vi "Get Zernike Coefficients 2.vi"(8 "error in (no error)":errorcluster, 9 "Pupil":cluster{"center":T2, "radius":sgl}, 10 "PupilDetectionOption":T1, 11 "HasoSlopes in":refnum<class "HasoSlopes.lvclass">) -> (0 "error out":errorcluster, 1 "Pupil out":cluster{"center":T2, "radius":sgl}, 2 "Zernike Coefficients":dbl[](array[numeric]), 3 "HasoSlopes out":refnum<class "HasoSlopes.lvclass">)   [LabVIEW 2020]
uses:
  WaveKit/Controls/Point2Df.ctl
  WaveKit/Controls/CircularPupilDetectionParams.ctl
  WaveKit/Controls/PupilDetectionOption.ctl
  WaveKit/Controls/CircularAutoDetectionOptions.ctl
  WaveKit/Controls/PupilDetectionMode.ctl
  WaveKit/Classes/HasoSlopes/HasoSlopes.lvclass
  WaveKit/Classes/ComputePhaseSet/ComputePhaseSet.lvclass
  WaveKit/Classes/Pupil/Pupil.lvclass
  WaveKit/Controls/ZernikeModalPrefs.ctl
  WaveKit/Controls/ZernikeProjectionPupilSetup.ctl
  WaveKit/Classes/ModalCoef/ModalCoef.lvclass
  WaveKit/Controls/WavefrontReconstructionMode.ctl
  WaveKit/Controls/WavefrontModalReconstructionType.ctl
  WaveKit/Classes/HasoData/HasoData.lvclass
panel:
  in  "CircularPupilDetectionParams":T3={"PupilDetectionOption"=enum."Automatic", "AutoDetectionOption"=enum."auto_radius_auto_center", "PupilDetectionMode"=enum."inscribed", "CentralOccultationDetection"=FALSE}
  out "radius":sgl
  out "center":T2
  out "Zernike pupil":i32[][](graph)
  out "Measured pupil":i32[][](graph)
  # "21.9945"
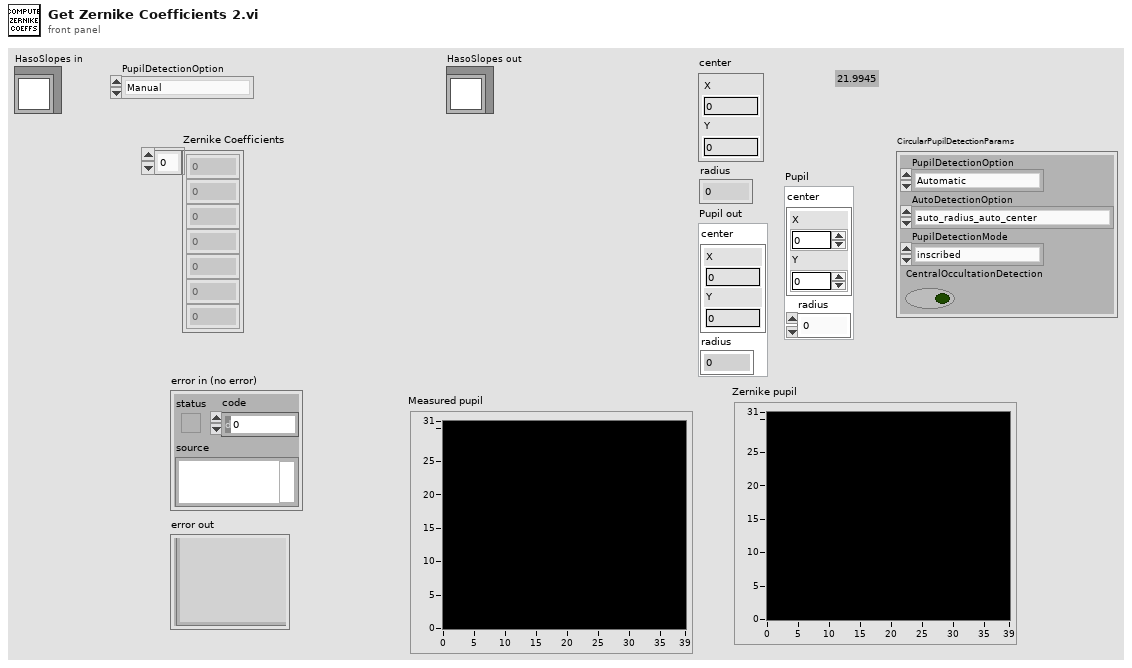
[diagram p1: front panel]
types:
  T1 = typedef "PupilDetectionOption.ctl" = enum16{"Manual", "Automatic"}
  T2 = typedef "Point2Df.ctl" = cluster{"X":sgl, "Y":sgl}
  T3 = typedef "CircularPupilDetectionParams.ctl" = cluster{"PupilDetectionOption":T1, "AutoDetectionOption":T4, "PupilDetectionMode":T5, "CentralOccultationDetection":bool}
  T4 = typedef "CircularAutoDetectionOptions.ctl" = enum16{"manual_radius_auto_center", "manual_center_auto_radius", "auto_radius_auto_center"}
  T5 = typedef "PupilDetectionMode.ctl" = enum16{"inscribed", "circumscribed"}
  T6 = typedef "WavefrontModalReconstructionType.ctl" = enum16{"Legendre", "Zernike"}
  T7 = typedef "WavefrontReconstructionMode.ctl" = enum16{"None", "Modal_Legendre", "Modal_Zernike", "Zonal", "Modal_Zonal_Zernike", "Modal_Zonal_Legendre"}
  T8 = typedef "ZernikeModalPrefs.ctl" = cluster{"Number of coefficients":u32, "Filtered coefficients":u32[], "RMS Zernike normalization":bool, "CircularProjectionPupilDimensions":T9}
  T9 = typedef "ZernikeProjectionPupilSetup.ctl" = cluster{"Pupil center_sspp":T2, "Pupil radius_sspp":sgl}
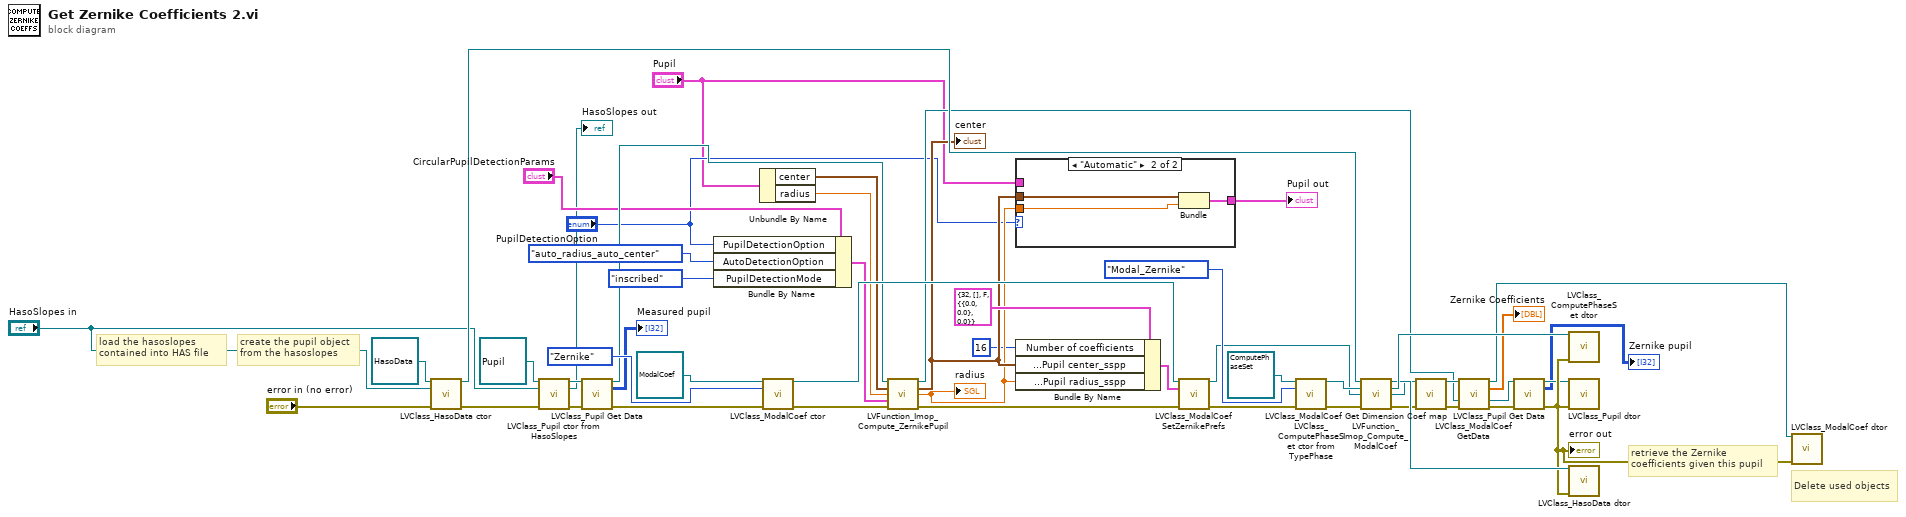
[diagram p0: block diagram]
diagram:
  # "Delete used objects"
  # "retrieve the Zernike\ncoefficients given this pupil"
  # "create the pupil object\nfrom the hasoslopes"
  # "load the hasoslopes\ncontained into HAS file"
  n1 = call "LVClass_HasoData ctor.vi"("HasoData (const)"=refnum<class "HasoData.lvclass"> refnum ("HasoData in"), "HasoSlopes"="HasoSlopes in", "error in (no error)"="error in (no error)") -> ("HasoData (new)"=w33:refnum<class "HasoData.lvclass">, "error out"=w31:errorcluster)  [unwired: 10 in, 1 out]
  n2 = call "LVClass_Pupil ctor from HasoSlopes.vi"("Pupil (const)"=refnum<class "Pupil.lvclass"> refnum ("Pupil in"), "HasoSlopes"="HasoSlopes in", "error in (no error)"=w31) -> ("Pupil (new)"=w29:refnum<class "Pupil.lvclass">, "HasoSlopes (dup)"=→"HasoSlopes out":refnum<class "HasoSlopes.lvclass">, "error out"=w27:errorcluster)  [unwired: 10 in]
  n3 = call "LVClass_Pupil Get Data.vi"("Pupil in"=w29, "error in (no error)"=w27) -> ("Pupil out"=w28:refnum<class "Pupil.lvclass">, "Data"=→"Measured pupil":i32[][], "error out"=w18:errorcluster)  [unwired: 11 in]
  n4 = Bundle By Name(cluster="CircularPupilDetectionParams", "PupilDetectionOption"="PupilDetectionOption", "AutoDetectionOption"=CircularAutoDetectionOptions."auto_radius_auto_center", "PupilDetectionMode"=PupilDetectionMode."inscribed") -> (w8:T3)
  n5 = Unbundle By Name("Pupil") -> ("center"=w15:T2, "radius"=w14:sgl)
  n6 = call "LVClass_ModalCoef ctor.vi"("ModalCoef (const)"=refnum<class "ModalCoef.lvclass"> refnum ("ModalCoef in"), "TypePhase"=WavefrontModalReconstructionType."Zernike", "error in (no error)"=w18) -> ("ModalCoef (new)"=w35:refnum<class "ModalCoef.lvclass">, "error out"=w30:errorcluster)  [unwired: 11 in]
  n7 = call "LVFunction_Imop_Compute_ZernikePupil.vi"("Pupil.lvclass"=w28, "center in"=w15, "radius in"=w14, "CircularPupilDetectionParams"=w8, "error in"=w30) -> ("Pupil.lvclass"=w24:refnum<class "Pupil.lvclass">, "center"=w13:T2, "radius"=w12:sgl, "error out"=w25:errorcluster)  [unwired: 7 in]
  "center" <- w13
  "radius" <- w12
  n8 = case shown="\"Automatic\"" "PupilDetectionOption" {
    tunnel: w13 -> [_ w55]
    tunnel: w12 -> [_ w54]
    tunnel: [w52 w53] -> w11
    tunnel: "Pupil" -> [w52 _]
    frame "Manual", Default {
    }
    frame "Automatic" {
      n9 = Bundle("center"=w55, "radius"=w54) -> (w53:cluster{"center":T2, "radius":sgl})  [unwired: 1 in]
    }
  }
  "Pupil out" <- w11
  n10 = Bundle By Name(cluster=T8 {"Number of coefficients"=32, "Filtered coefficients"=[], "RMS Zernike normalization"=FALSE, "CircularProjectionPupilDimensions"={"Pupil center_sspp"={"X"=0.0, "Y"=0.0}, "Pupil radius_sspp"=0.0}} ("ZernikeModalPrefs"), "Number of coefficients"=u32 16, "CircularProjectionPupilDimensions.Pupil center_sspp"=w13, "CircularProjectionPupilDimensions.Pupil radius_sspp"=w12) -> (w41:T8)
  n11 = call "LVClass_ModalCoef SetZernikePrefs.vi"("ModalCoef in"=w35, "ZernikeModalPrefs"=w41, "error in (no error)"=w25) -> ("ModalCoef out"=w36:refnum<class "ModalCoef.lvclass">, "error out"=w17:errorcluster)  [unwired: 11 in]
  n12 = call "LVClass_ComputePhaseSet ctor from TypePhase.vi"("ComputePhaseSet (const)"=refnum<class "ComputePhaseSet.lvclass"> refnum ("ComputePhaseSet in"), "TypePhase"=WavefrontReconstructionMode."Modal_Zernike", "error in (no error)"=w17) -> ("ComputePhaseSet (new)"=w37:refnum<class "ComputePhaseSet.lvclass">, "error out"=w16:errorcluster)  [unwired: 11 in]
  n13 = call "LVFunction_Imop_Compute_ModalCoef.vi"("HasoData.lvclass"=w33, "ComputePhaseSet.lvclass"=w37, "ModalCoef.lvclass"=w36, "error constant"=w16) -> ("HasoData.lvclass (dup)"=w46:refnum<class "HasoData.lvclass">, "ComputePhaseSet.lvclass (dup)"=w47:refnum<class "ComputePhaseSet.lvclass">, "ModalCoef.lvclass (dup)"=w32:refnum<class "ModalCoef.lvclass">, "error out"=w43:errorcluster)  [unwired: 8 in]
  n14 = call "LVClass_ModalCoef Get Dimension Coef map.vi"("ModalCoef in"=w32, "error in (no error)"=w43) -> ("ModalCoef out"=w48:refnum<class "ModalCoef.lvclass">, "error out"=w44:errorcluster)  [unwired: 11 in, 1 out]
  n15 = call "LVClass_ModalCoef GetData.vi"("ModalCoef in"=w48, "Pupil.lvclass"=w24, "error in (no error)"=w44) -> ("ModalCoef out"=w45:refnum<class "ModalCoef.lvclass">, "coef"=→"Zernike Coefficients":sgl[], "Pupil.lvclass (dup)"=w23:refnum<class "Pupil.lvclass">, "error out"=w22:errorcluster)  [unwired: 8 in, 1 out]
  n16 = call "LVClass_Pupil Get Data.vi"("Pupil in"=w23, "error in (no error)"=w22) -> ("Pupil out"=w20:refnum<class "Pupil.lvclass">, "Data"=→"Zernike pupil":i32[][], "error out"=w21:errorcluster)  [unwired: 11 in]
  "error out" <- w21
  n17 = call "LVClass_ComputePhaseSet dtor.vi"("ComputePhaseSet in"=w47, "error in (no error)"=w21) -> ()  [unwired: 12 in, 2 out]
  n18 = call "LVClass_Pupil dtor.vi"("Pupil in"=w20, "error in (no error)"=w21) -> ()  [unwired: 12 in, 2 out]
  n19 = call "LVClass_HasoData dtor.vi"("HasoData in"=w46, "error in (no error)"=w21) -> ()  [unwired: 12 in, 2 out]
  n20 = call "LVClass_ModalCoef dtor.vi"("ModalCoef in"=w45, "error in (no error)"=w21) -> ()  [unwired: 12 in, 2 out]
